vi "test-Encrypt (FFT).vi"(8 "error in (no error)":errorcluster, 11 "TestCase in":refnum<class "Test-Encryption.lvclass">=refnum) -> (0 "error out":errorcluster, 3 "TestCase out":refnum<class "Test-Encryption.lvclass">)   [LabVIEW 2019, in "Test-Encryption.lvclass"]
uses:
  Test-Encryption.lvclass
  Encryption/Encryption.lvclass
  Encryption/FFT/FFT.lvclass
  Layouts/Layout.lvclass
  C:/Development/Open Source/tsc-event-logger/Encryption/Encryption.lvclass
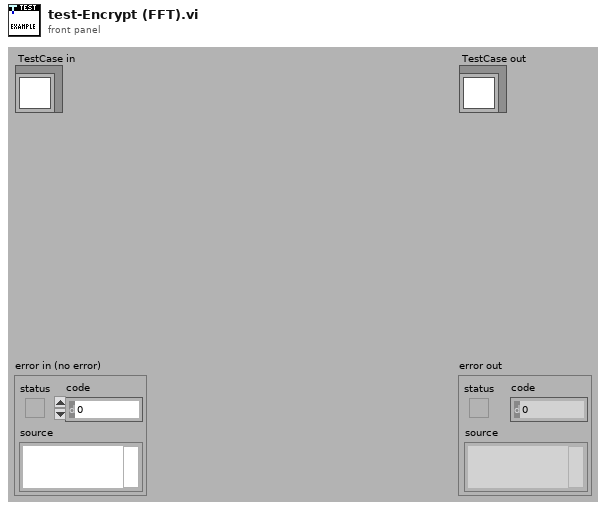
[diagram p1: front panel]
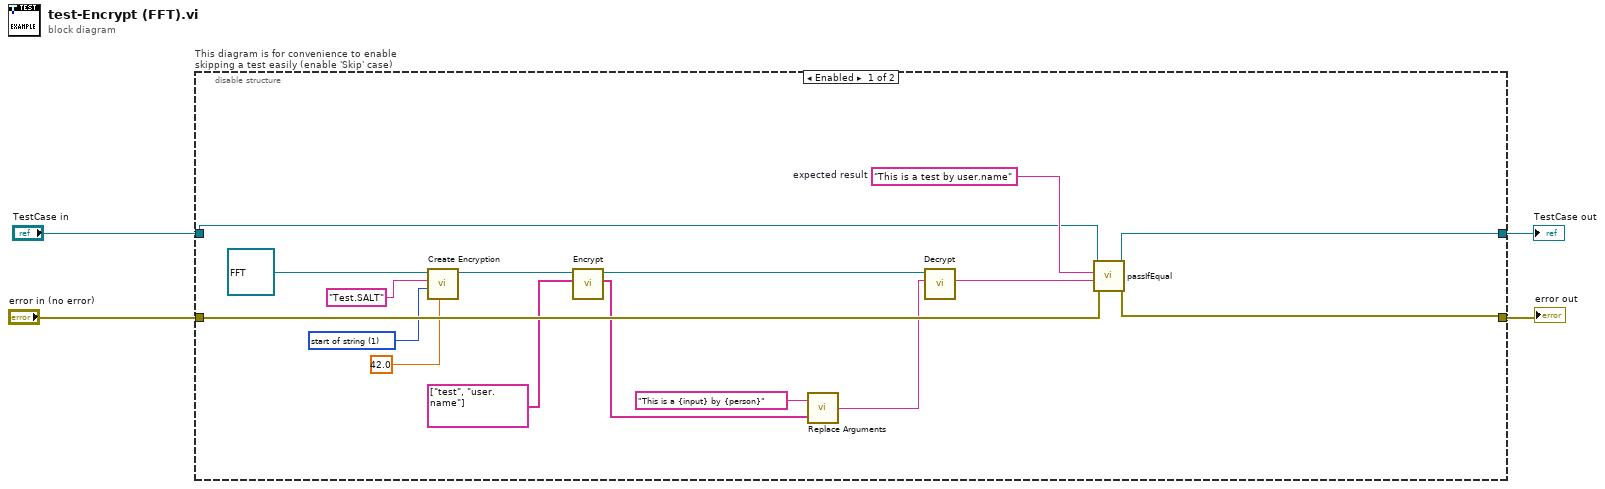
[diagram p0: block diagram]
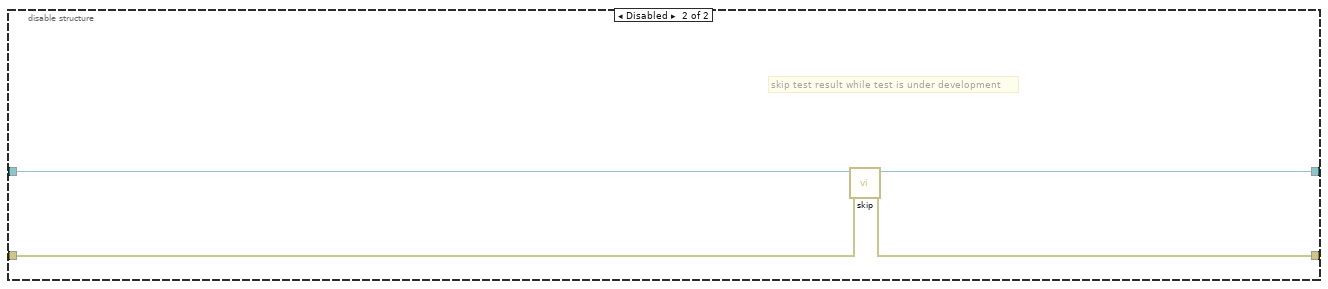
[diagram p2: hidden frame]
diagram:
  n1 = disable-structure "This diagram is for convenience to enable skipping a test easily (enable 'Skip' case)" shown="Enabled" {
    disable-tunnel: "TestCase in" -> [w19 w24]
    disable-tunnel: [w18 w22] -> w1
    disable-tunnel: [w17 w23] -> w3
    disable-tunnel: "error in (no error)" -> [w16 w21]
    frame Enabled {
      w13 = u16 1 items=["both", "start of string", "end of string"] ("SALT location (start of string)")
      w20 = "This is a test by user.name"  # expected result
      n2 = call "Create Encryption.vi"("Multiplier"=42.0, "SALT location (start of string)"=w13, "SALT"="Test.SALT", "Encryption Method"=refnum<class "FFT.lvclass"> refnum ("TSC Event Logger.lvlib:FFT.lvclass")) -> ("Encryption output"=w11:refnum<class "FFT.lvclass">)  [unwired: 6 in, 1 out]
      n3 = call-dynamic "Encrypt.vi"("Arguments"=string[] ["test", "user.name"], "FFT in"=w11) -> ("Encrypted Arguments"=w7:string[], "FFT out"=w8:refnum<class "FFT.lvclass">)  [unwired: 7 in, 1 out]
      n4 = call "Replace Arguments.vi"("Arguments"=w7, "Message"="This is a {input} by {person}") -> ("Output Message"=w6:string)
      n5 = call-dynamic "Decrypt.vi"("Message"=w6, "FFT in"=w8) -> ("Decrypted Message"=w5:string)  [unwired: 7 in, 2 out]
      n6 = call-dynamic "passIfEqual.vi"("error in (no error)"=w16, "y"=w5, "x"=w20, "TestCase in"=w19) -> ("error out"=w17:errorcluster, "TestCase out"=w18:refnum<class "Test-Encryption.lvclass">)  [unwired: 6 in]
    }
    frame Disabled {
      # "skip test result while test is under development"
      n7 = call <vilib>:"skip.vi"("error in (no error)"=w21, "TestCase in"=w24) -> ("error out"=w23:errorcluster, "TestCase out"=w22:refnum<class "Test-Encryption.lvclass">)  [unwired: 8 in]
    }
  }
  "error out" <- w3
  "TestCase out" <- w1
